vi "Dis_Number_Fixture.vi"(8 "Lane Tyep":string(combo)="[_]", 11 "Fixture_Data":u16[](array[numeric])) -> (0 "Color Master Unit":u32(colorbox), 1 "Color Result":u32(colorbox), 2 "Lane Number":string, 3 "Product Number":string, 5 "Zero":bool)   [LabVIEW 2017]
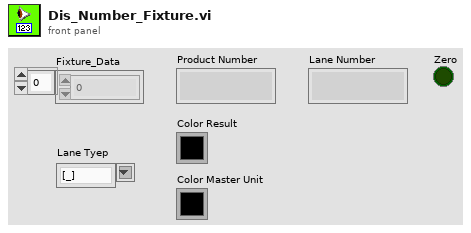
[diagram p1: front panel]
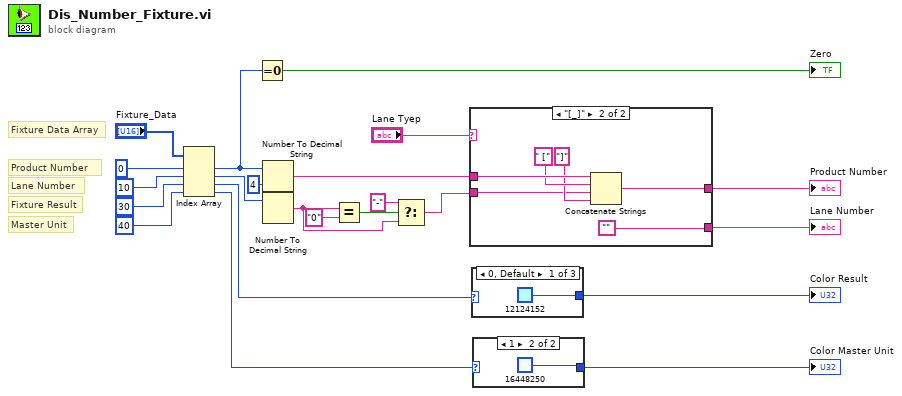
[diagram p0: block diagram]
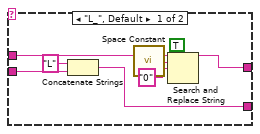
[diagram p2: hidden frame]
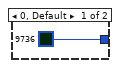
[diagram p3: hidden frame]
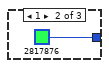
[diagram p4: hidden frame]
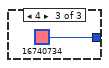
[diagram p5: hidden frame]
diagram:
  # "Master Unit"
  # "Fixture Result"
  # "Fixture Data Array"
  # "Lane Number"
  # "Product Number"
  n1 = Index Array(array="Fixture_Data", index #1=0 ("index"), index #2=10 ("index"), index #3=30 ("index"), index #4=40 ("index")) -> (element #1=w2:u16, element #2=w19:u16, element #3=w15:u16, element #4=w7:u16)
  n2 = Equal To 0?(x=w2) -> (x = 0?=→"Zero":bool)
  n3 = Number To Decimal String(number=w2, width (-)=i16 4) -> (decimal integer string=w18:string)
  n4 = Number To Decimal String(number=w19) -> (decimal integer string=w10:string)  [unwired: 1 in]
  n5 = Equal?(x=w10, y="0") -> (x = y?=w12:bool)
  n6 = Select(t="-", s=w12, f=w10) -> (s? t:f=w9:string)
  n7 = case shown="\"[_]\"" "Lane Tyep" {
    tunnel: w18 -> [w24 w36]
    tunnel: [w23 w34] -> w17
    tunnel: w9 -> [w29 w32]
    tunnel: [w28 ""] -> w4
    frame "L_", Default {
      n8 = Concatenate Strings("L" ("string"), w29) -> (w28:string)
      n9 = call <vilib>:"Space Constant.vi"() -> ("String"=w27:string)
      n10 = Search and Replace String(replace all?=TRUE ("replace all? (F)"), input string=w24, search string=w27, replace string="0" ("replace string (\"\")")) -> (result string=w23:string)  [unwired: 4 in, 3 out]
    }
    frame "[_]" {
      n11 = Concatenate Strings(w36, " [" ("string"), w32, "]" ("string")) -> (w34:string)
    }
  }
  "Product Number" <- w17
  "Lane Number" <- w4
  n12 = case shown="0, Default" w15 {
    tunnel: [u32 12124152 u32 2817876 u32 16740734] -> w14
    frame 0, Default {
    }
    frame 1 {
    }
    frame 4 {
    }
  }
  "Color Result" <- w14
  n13 = case shown="1" w7 {
    tunnel: [u32 9736 u32 16448250] -> w6
    frame 0, Default {
    }
    frame 1 {
    }
  }
  "Color Master Unit" <- w6
